vi "Cage_setup_171213.vi"(6 "Close port? (T)":bool, 8 "VISA resource name":refnum<visa-resource-name>="ASRL3::INSTR") -> (0 "Record_flag":refnum<notifier>, 1 "error":bool, 2 "ReadStatus":refnum<notifier>, 3 "VISA resource name out":refnum<visa-resource-name>)   [LabVIEW 2016]
uses:
  <vilib>/Instr/_visa.llb/VISA Set IO Buffer Mask.ctl
  <vilib>/Instr/_visa.llb/VISA Configure Serial Port (Instr).vi
  Globaltracker.vi
panel:
  out "error out 2":errorcluster
  out "read buffer":string
  out "Poll Binary":u32
  out "Poll Matrix":u32
  out "Poll Coord":u32
  out "Poll FPS":u32
  out "FPS status":i32
  out "Matrix mode status":string
  out "Coordinate mode status":string
  out "Binary mode status":string
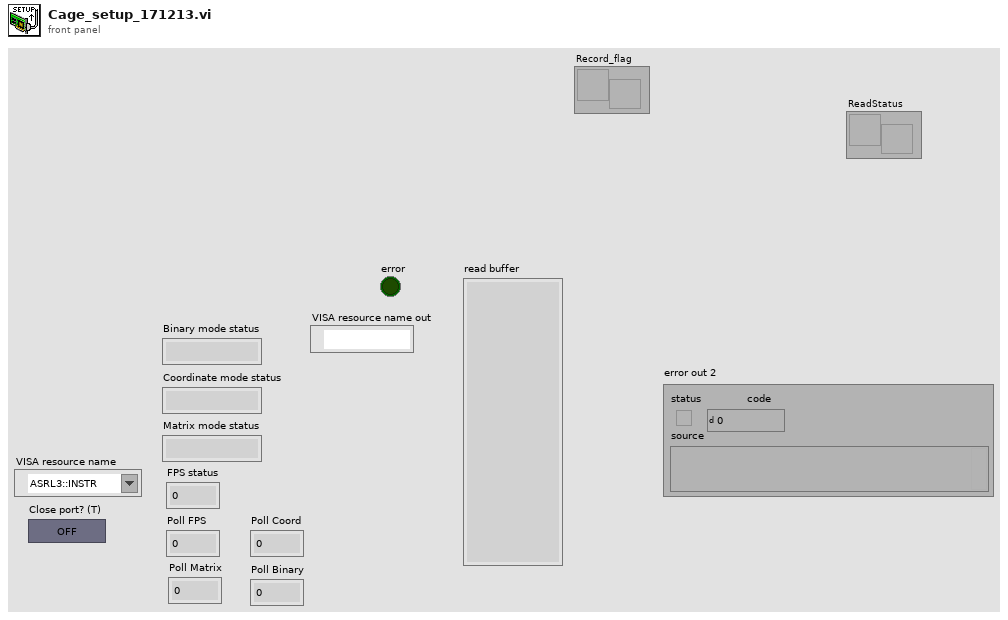
[diagram p1: front panel]
types:
  T1 = typedef "VISA Set IO Buffer Mask.ctl" = u16
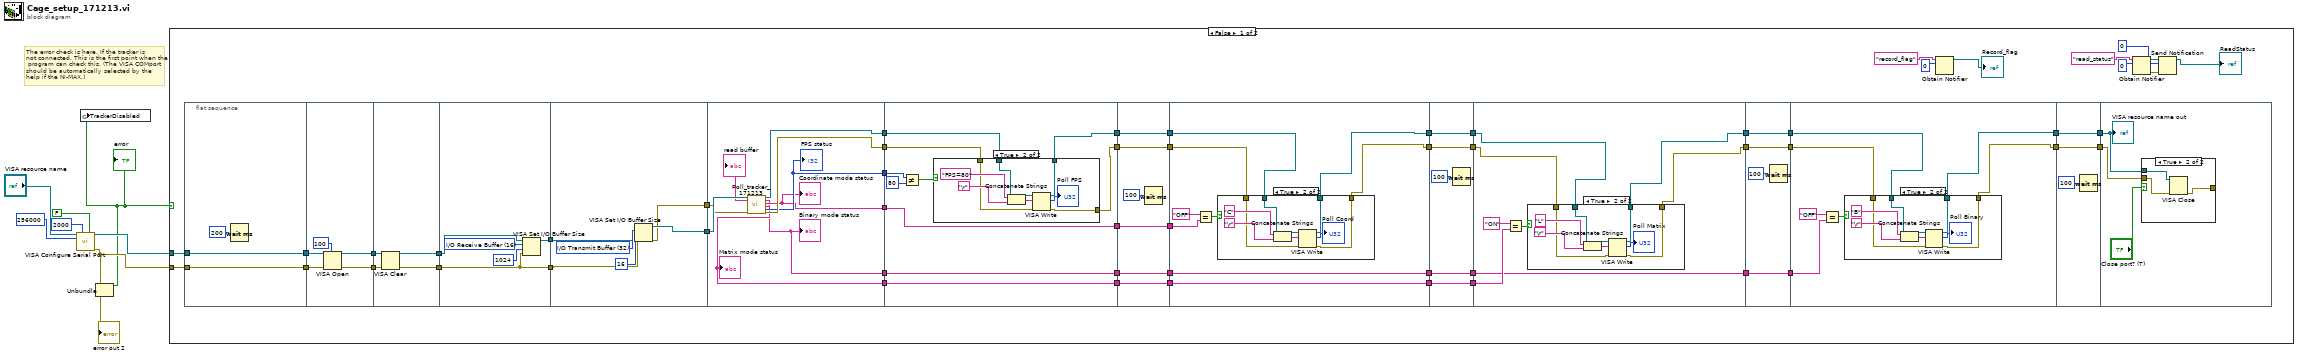
[diagram p0: block diagram]
diagram:
  # "The error check is here. If the tracker is \nnot connected. This is the first point when the\n program can check this. (The VISA COMport \nshould be automatically selected by the \nhelp if the NI-MAX.)"
  n1 = call-poly "VISA Configure Serial Port"("VISA resource name"="VISA resource name", "timeout (10sec)"=u32 2000, "Enable Termination\nChar (T)"=FALSE ("Enable Termination\nChar (T)"), "baud rate (9600)"=u32 256000) -> ("VISA resource name out"=w3:refnum<visa-resource-name>, "error out"=w2:errorcluster)  [unwired: 10 in]
  "error out 2" <- w2
  n2 = Unbundle(w2) -> ("status"=w1:bool)  [unwired: 2 out]
  "error" <- w1
  n3 = global write "Globaltracker.vi" "TrackerDisabled"(w1) -> ()
  n4 = case shown="False" w1 {
    tunnel: w3 -> [w18 _]
    tunnel: w2 -> [w17 _]
    frame False {
      n5 = flat-sequence {
        tunnel: [w64] -> w62
        tunnel: [w63] -> w61
        tunnel: w18 -> [w64]
        tunnel: w17 -> [w63]
        tunnel: w62 -> [w68]
        tunnel: [w67] -> w59
        tunnel: w61 -> [w70]
        tunnel: [w69] -> w60
        tunnel: w60 -> [w73]
        tunnel: w59 -> [w74]
        tunnel: [w72] -> w58
        tunnel: [w71] -> w57
        tunnel: [w75] -> w55
        tunnel: [w79] -> w56
        tunnel: w58 -> [w75]
        tunnel: w57 -> [w77]
        tunnel: w56 -> [w83]
        tunnel: [w82] -> w54
        tunnel: w55 -> [w81]
        tunnel: [w80] -> w53
        tunnel: [w91] -> w51
        tunnel: [w92] -> w52
        tunnel: w54 -> [w94]
        tunnel: w53 -> [w93]
        tunnel: [w90] -> w50
        tunnel: [w89] -> w49
        tunnel: [w88] -> w48
        tunnel: [w87] -> w47
        tunnel: w52 -> [w101]
        tunnel: [w98] -> w46
        tunnel: w51 -> [w100]
        tunnel: [w99] -> w45
        tunnel: w50 -> [w103]
        tunnel: [w97] -> w44
        tunnel: w49 -> [w97]
        tunnel: [w96] -> w43
        tunnel: w48 -> [w96]
        tunnel: [w95] -> w42
        tunnel: w47 -> [w95]
        tunnel: w46 -> [w120]
        tunnel: [w120] -> w41
        tunnel: w45 -> [w119]
        tunnel: [w119] -> w40
        tunnel: [w117] -> w39
        tunnel: w44 -> [w117]
        tunnel: [w116] -> w38
        tunnel: w43 -> [w116]
        tunnel: [w115] -> w37
        tunnel: w42 -> [w115]
        tunnel: w41 -> [w128]
        tunnel: [w126] -> w36
        tunnel: w40 -> [w127]
        tunnel: [w123] -> w35
        tunnel: w39 -> [w125]
        tunnel: w38 -> [w122]
        tunnel: [w122] -> w34
        tunnel: w37 -> [w121]
        tunnel: [w121] -> w33
        tunnel: w36 -> [w144]
        tunnel: [w144] -> w32
        tunnel: w35 -> [w143]
        tunnel: [w143] -> w31
        tunnel: [w141] -> w30
        tunnel: w34 -> [w141]
        tunnel: [w140] -> w29
        tunnel: w33 -> [w140]
        tunnel: w32 -> [w150]
        tunnel: [w148] -> w28
        tunnel: w31 -> [w149]
        tunnel: [w147] -> w27
        tunnel: w30 -> [w146]
        tunnel: w29 -> [w145]
        tunnel: [w145] -> w26
        tunnel: w28 -> [w166]
        tunnel: [w166] -> w25
        tunnel: w27 -> [w165]
        tunnel: [w165] -> w24
        tunnel: [w163] -> w23
        tunnel: w26 -> [w163]
        tunnel: w25 -> [w171]
        tunnel: [w169] -> w22
        tunnel: w24 -> [w170]
        tunnel: [w168] -> w21
        tunnel: w23 -> [w167]
        tunnel: w22 -> [w186]
        tunnel: [w186] -> w20
        tunnel: [w185] -> w19
        tunnel: w21 -> [w185]
        tunnel: w20 -> [w188]
        tunnel: w19 -> [w189]
        frame #0 {
          n6 = Wait (ms)(milliseconds to wait=u32 200) -> ()  [unwired: 1 out]
        }
        frame #1 {
          n7 = VISA Open(timeout (0)=u32 100 ("VISA Open timeout (0)"), error in (no error)=w70, VISA resource name=w68) -> (VISA resource name=w67:refnum<visa-resource-name>, error out=w69:errorcluster)  [unwired: 2 in]
        }
        frame #2 {
          n8 = VISA Clear(VISA resource name=w74, error in (no error)=w73) -> (VISA resource name out=w71:refnum<visa-resource-name>, error out=w72:errorcluster)
        }
        frame #3 {
          w76 = T1 16 items=["I/O Receive Buffer"=16, "I/O Transmit Buffer"=32, "I/O Receive and Transmit Buffer"=48] ("Mask")
          n9 = VISA Set I/O Buffer Size(VISA resource name=w77, mask (16)=w76, size (4096)=u32 1024, error in (no error)=w75) -> (VISA resource name out=w79:refnum<visa-resource-name>)  [unwired: 1 out]
        }
        frame #4 {
          w84 = T1 32 items=["I/O Receive Buffer"=16, "I/O Transmit Buffer"=32, "I/O Receive and Transmit Buffer"=48] ("Mask")
          n10 = VISA Set I/O Buffer Size(VISA resource name=w83, mask (16)=w84, size (4096)=u32 16, error in (no error)=w81) -> (VISA resource name out=w82:refnum<visa-resource-name>, error out=w80:errorcluster)
        }
        frame #5 {
          n11 = call "Poll_tracker_171213.vi"("VISA resource name"=w94, "error in (no error)"=w93) -> ("read buffer"=→"read buffer":string, "VISA resource name out"=w92:refnum<visa-resource-name>, "Binary mode status"=w87:string, "Coordinate mode status"=w89:string, "Matrix mode status"=w88:string, "FPS status"=w90:i32, "error out"=w91:errorcluster)  [unwired: 11 in]
          "Binary mode status" <- w87
          "Coordinate mode status" <- w89
          "Matrix mode status" <- w88
          "FPS status" <- w90
        }
        frame #6 {
          n12 = Not Equal?(x=w103, y=80) -> (x != y?=w104:bool)
          n13 = case shown="True" w104 {
            tunnel: w101 -> [w106 w110]
            tunnel: w100 -> [w105 w109]
            tunnel: [w105 w108] -> w99
            tunnel: [w106 w107] -> w98
            frame False {
            }
            frame True {
              n14 = Concatenate Strings("FPS=80" ("write buffer"), "\r") -> (w112:string)
              n15 = VISA Write(VISA resource name=w110, write buffer=w112, error in (no error)=w109) -> (VISA resource name out=w107:refnum<visa-resource-name>, return count=→"Poll FPS":u32, error out=w108:errorcluster)
            }
          }
        }
        frame #7 {
          n16 = Wait (ms)(milliseconds to wait=u32 100) -> ()  [unwired: 1 out]
        }
        frame #8 {
          n17 = Equal?(x="OFF", y=w125) -> (x = y?=w129:bool)
          n18 = case shown="True" w129 {
            tunnel: w128 -> [w131 w135]
            tunnel: w127 -> [w130 w134]
            tunnel: [w131 w133] -> w126
            tunnel: [w130 w132] -> w123
            frame False {
            }
            frame True {
              n19 = Concatenate Strings("C" ("write buffer"), "\r") -> (w137:string)
              n20 = VISA Write(VISA resource name=w135, write buffer=w137, error in (no error)=w134) -> (VISA resource name out=w133:refnum<visa-resource-name>, return count=→"Poll Coord":u32, error out=w132:errorcluster)
            }
          }
        }
        frame #9 {
          n21 = Wait (ms)(milliseconds to wait=u32 100) -> ()  [unwired: 1 out]
        }
        frame #10 {
          n22 = Equal?(x="ON", y=w146) -> (x = y?=w152:bool)
          n23 = case shown="True" w152 {
            tunnel: w150 -> [w154 w158]
            tunnel: w149 -> [w153 w157]
            tunnel: [w154 w156] -> w148
            tunnel: [w153 w155] -> w147
            frame False {
            }
            frame True {
              n24 = Concatenate Strings("L" ("write buffer"), "\r") -> (w160:string)
              n25 = VISA Write(VISA resource name=w158, write buffer=w160, error in (no error)=w157) -> (VISA resource name out=w156:refnum<visa-resource-name>, return count=→"Poll Matrix":u32, error out=w155:errorcluster)
            }
          }
        }
        frame #11 {
          n26 = Wait (ms)(milliseconds to wait=u32 100) -> ()  [unwired: 1 out]
        }
        frame #12 {
          n27 = Equal?(x="OFF", y=w167) -> (x = y?=w173:bool)
          n28 = case shown="True" w173 {
            tunnel: w171 -> [w175 w179]
            tunnel: w170 -> [w174 w178]
            tunnel: [w175 w177] -> w169
            tunnel: [w174 w176] -> w168
            frame False {
            }
            frame True {
              n29 = Concatenate Strings("B" ("write buffer"), "\r") -> (w181:string)
              n30 = VISA Write(VISA resource name=w179, write buffer=w181, error in (no error)=w178) -> (VISA resource name out=w177:refnum<visa-resource-name>, return count=→"Poll Binary":u32, error out=w176:errorcluster)
            }
          }
        }
        frame #13 {
          n31 = Wait (ms)(milliseconds to wait=u32 100) -> ()  [unwired: 1 out]
        }
        frame #14 {
          n32 = case shown="True" "Close port? (T)" {
            tunnel: w189 -> [w190 w193]
            tunnel: [w190 w192] -> _
            tunnel: w188 -> [_ w191]
            frame False {
            }
            frame True {
              n33 = VISA Close(VISA resource name=w191, error in (no error)=w193) -> (error out=w192:errorcluster)
            }
          }
          "VISA resource name out" <- w188
        }
      }
      n34 = Obtain Notifier(name (unnamed)="record_flag", notification data type=0) -> (notifier out=→"Record_flag":refnum<notifier>)  [unwired: 2 in, 2 out]
      n35 = Obtain Notifier(name (unnamed)="read_status", notification data type=0) -> (notifier out=w12:refnum<notifier>, error out=w13:errorcluster)  [unwired: 2 in, 1 out]
      n36 = Send Notification(notification=0, notifier=w12, error in (no error)=w13) -> (notifier out=→"ReadStatus":refnum<notifier>)  [unwired: 1 out]
    }
    frame True {
    }
  }
